vi "VI Tree - Msg Queue__ogtk.vi"() -> ()   [LabVIEW 2017]
uses:
  <userlib>/_OpenG.lib/msgqueue/msgqueue.llb/Msg Cluster__ogtk.ctl
  <userlib>/_OpenG.lib/msgqueue/msgqueue.llb/Msg Queue RefNum__ogtk.ctl
panel:
  in  "Case Constant\n(See Context Help)":bool
  out "msg queue":T1
  out "message cluster":T2
  # "[OpenG VI Tags] ***Do Not Remove***"
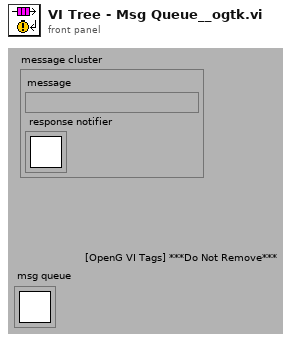
[diagram p1: front panel]
types:
  T1 = typedef "Msg Queue RefNum__ogtk.ctl" = refnum<k1>
  T2 = typedef "Msg Cluster__ogtk.ctl" = cluster{"message":string, "response notifier":T3}
  T3 = typedef "Notifier RefNum" = refnum<k1>
  T4 = typedef "Queue RefNum" = refnum<k1>
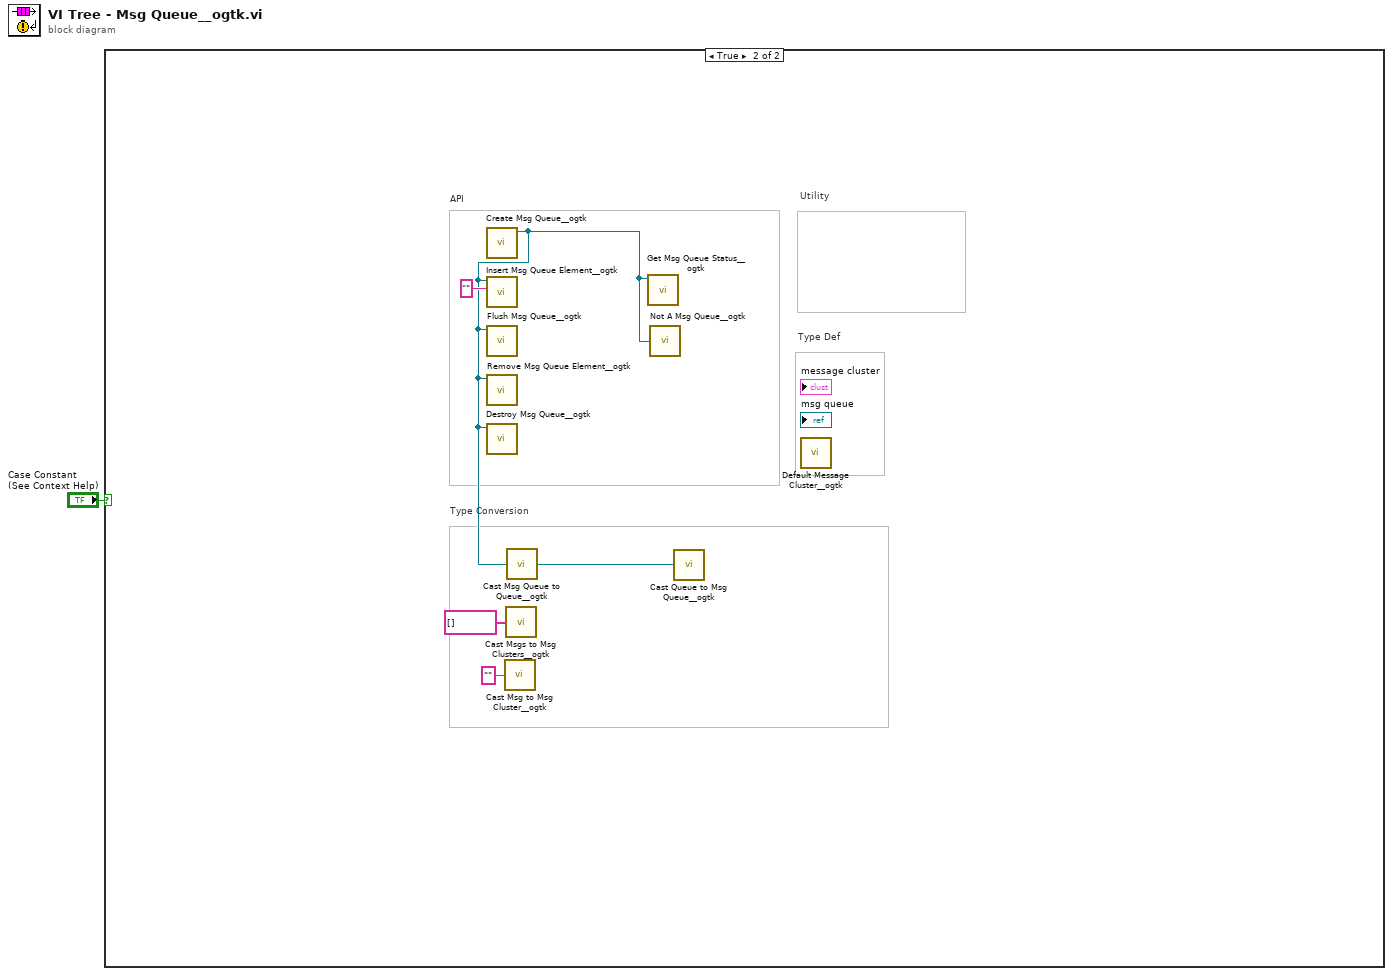
[diagram p0: block diagram]
diagram:
  n1 = case shown="True" "Case Constant\n(See Context Help)" {
    frame False {
    }
    frame True {
      # "Type Def"
      # "Type Conversion"
      # "Utility"
      # "API"
      n2 = call <userlib>:"Create Msg Queue__ogtk.vi"() -> ("msg queue"=w2:T1)  [unwired: 5 in, 2 out]
      n3 = call <userlib>:"Insert Msg Queue Element__ogtk.vi"("message"="", "msg queue"=w2) -> ()  [unwired: 4 in, 4 out]
      n4 = call <userlib>:"Flush Msg Queue__ogtk.vi"("msg queue"=w2) -> ()  [unwired: 4 in, 3 out]
      n5 = call <userlib>:"Remove Msg Queue Element__ogtk.vi"("msg queue"=w2) -> ()  [unwired: 7 in, 4 out]
      n6 = call <userlib>:"Destroy Msg Queue__ogtk.vi"("msg queue"=w2) -> ()  [unwired: 4 in, 3 out]
      n7 = call <userlib>:"Cast Msg to Msg Cluster__ogtk.vi"("queue element"="") -> ()  [unwired: 4 in, 1 out]
      n8 = call <userlib>:"Cast Msgs to Msg Clusters__ogtk.vi"("queue elements"=string[] []) -> ()  [unwired: 4 in, 1 out]
      n9 = call <userlib>:"Cast Msg Queue to Queue__ogtk.vi"("msg queue"=w2) -> ("queue"=w5:T4)  [unwired: 4 in]
      n10 = call <userlib>:"Get Msg Queue Status__ogtk.vi"("msg queue"=w2) -> ()  [unwired: 3 in, 8 out]
      n11 = call <userlib>:"Not A Msg Queue__ogtk.vi"("msg queue"=w2) -> ()  [unwired: 1 out]
      n12 = call <userlib>:"Cast Queue to Msg Queue__ogtk.vi"("queue"=w5) -> ()  [unwired: 4 in, 1 out]
      n13 = call <userlib>:"Default Message Cluster__ogtk.vi"() -> ()  [unwired: 5 in, 1 out]
    }
  }
